vi "Demo - Transient Capture.vi"() -> ()   [LabVIEW 2017]
uses:
  Communications/Communications Library.lvlib
panel:
  in  "ARM":bool
  in  "Soft Trigger":bool=TRUE
  out "Waveform Graph":i16[][](graph)
  in  "configuration file path":path
  in  "Pre-Trigger Samples":i32
  in  "Post-Trigger Samples":i32
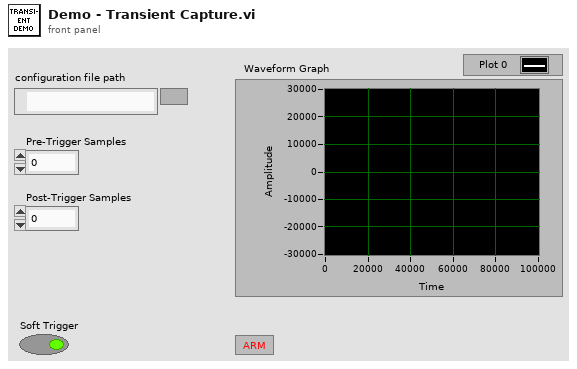
[diagram p1: front panel]
types:
  T1 = typedef "Communications Library.lvlib/DTACQ Module Carrier Configuration--Cluster.ctl" = cluster{"Name":string, "IP":string, "Control Port":i32, "Timeout (ms)":i32, "Continuous Capture Port (Multiplexed)":i32, "Start HIL Shot Port":i32, "AWG Upload Port (Multiplexed)":i32, "Download Captured Data Port (Multiplexed)":i32, "Module Slots":i32, "Module Configurations":T2[]}
  T2 = typedef "Communications Library.lvlib/DTACQ Module Configuration--Cluster.ctl" = cluster{"Name":string, "Position":string, "Module Type":T3, "Control Port":i32, "Timeout (ms)":i32, "Channels":i32}
  T3 = typedef "Communications Library.lvlib/DTACQ Device Type--Enum.ctl" = enum16{"Carrier", "Analog In Module", "Analog Out Module", "Generic Module"}
  T4 = typedef "Communications Library.lvlib/DTACQ Connection Data--Cluster.ctl" = cluster{"Description":string, "Address":string, "Port":u16, "timeout (ms)":i32, "Termination Character":string, "TCP Connection Reference":refnum<k5>, "Open Connection":bool}
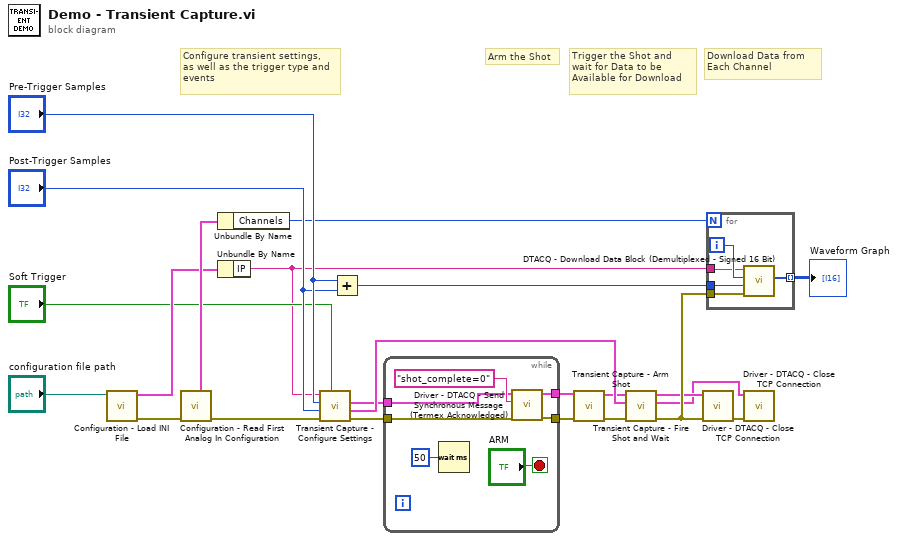
[diagram p0: block diagram]
diagram:
  # "Configure transient settings,\nas well as the trigger type and\nevents"
  # "Trigger the Shot and\nwait for Data to be\nAvailable for Download"
  # "Download Data from \nEach Channel"
  # "Arm the Shot"
  n1 = call "Configuration - Load INI File.vi"("configuration file path"="configuration file path") -> ("error out"=w18:errorcluster, "Carrier Configuration Out"=w16:T1)  [unwired: 9 in]
  n2 = call "Configuration - Read First Analog In Configuration.vi"("error in"=w18) -> ("error out"=w17:errorcluster, "AI - Module Configuration"=w19:T2)  [unwired: 6 in, 3 out]
  n3 = Unbundle By Name(w19) -> ("Channels"=w3:i32)
  n4 = Unbundle By Name(w16) -> ("IP"=w11:string)
  n5 = call "Transient Capture - Configure Settings.vi"("Soft Trigger"="Soft Trigger", "error in"=w17, "Samples to Read (Post Trigger)"="Post-Trigger Samples", "Samples to Read (Pre Trigger)"="Pre-Trigger Samples", "Address"=w11) -> ("error out"=w14:errorcluster, "AI Connection Out"=w7:T4, "Carrier Connection Out"=w2:T4)  [unwired: 4 in]
  n6 = Add(x="Pre-Trigger Samples", y="Post-Trigger Samples") -> (x+y=w10:i32)
  n7 = while {
    tunnel: w14 -> [w28]
    tunnel: [w27] -> w13
    tunnel: w2 -> [w26]
    tunnel: [w25] -> w1
    stop <- "ARM" stop-if-true
    n8 = Wait (ms)(milliseconds to wait=u32 50) -> ()  [unwired: 1 out]
    n9 = call "Driver - DTACQ - Send Synchronous Message (Termex Acknowledged).vi"("error in"=w28, "Message to Send"="shot_complete=0", "DTACQ Connection Data In"=w26) -> ("error out"=w27:errorcluster, "DTACQ Connection Data Out"=w25:T4)  [unwired: 5 in, 2 out]
  }
  n10 = call "Transient Capture - Arm Shot.vi"("error in"=w13, "Carrier Connection Out"=w1) -> ("error out"=w12:errorcluster, "DTACQ Connection Out"=w6:T4)  [unwired: 8 in]
  n11 = call "Transient Capture - Fire Shot and Wait.vi"("error in"=w12, "AI Connection In"=w7, "Carrier Connection In"=w6) -> ("error out"=w9:errorcluster, "AI Connection Out"=w4:T4, "Carrier Connection Out"=w5:T4)  [unwired: 6 in]
  n12 = call "Driver - DTACQ - Close TCP Connection.vi"("error in"=w9, "DTACQ Connection Data In"=w5) -> ("error out"=w8:errorcluster)  [unwired: 8 in, 1 out]
  n13 = for {
    N: w3 -> [_]
    tunnel: [w34] -> w20 mode=indexing
    tunnel: w10 -> [w33]
    tunnel: w11 -> [w32]
    tunnel: w9 -> [w31]
    i -> [w35]
    n14 = call "DTACQ - Download Data Block (Demultiplexed - Signed 16 Bit).vi"("error in"=w31, "Maximum Number of Samples"=w33, "Channel Number"=w35, "Address"=w32) -> ("(Signed) 16 Bit Array"=w34:i16[])  [unwired: 5 in, 2 out]
  }
  "Waveform Graph" <- w20
  n15 = call "Driver - DTACQ - Close TCP Connection.vi"("error in"=w8, "DTACQ Connection Data In"=w4) -> ()  [unwired: 8 in, 2 out]
